vi "validate.vi"(8 "error in":errorcluster, 11 "fixed channel configuration in":refnum<class "control module configuration.lvclass">) -> (0 "error out":errorcluster, 3 "fixed channel configuration out":refnum<class "control module configuration.lvclass">)   [LabVIEW 2013, in "control module configuration.lvclass"]
doc: "This function performs validation of the configuration. This function should be safe to call at any point and should not rely on anything in the runtime environment."
uses:
  control module configuration.lvclass
  <vilib>/NI/Tag Bus Module Framework/module configuration/TBM module configuration.lvclass
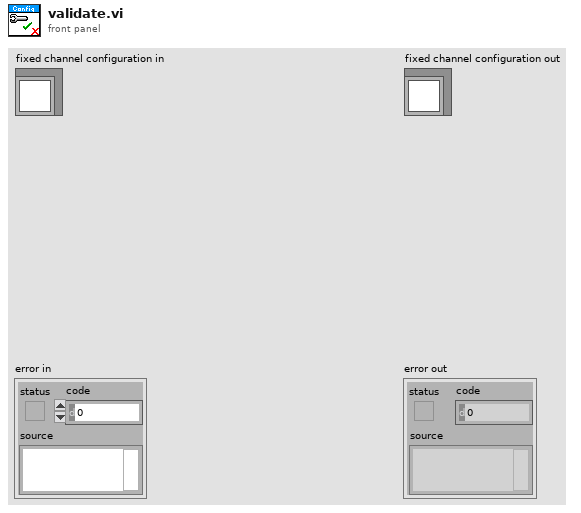
[diagram p1: front panel]
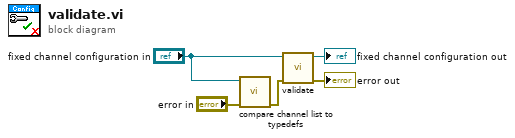
[diagram p0: block diagram]
diagram:
  n1 = call "compare channel list to typedefs.vi"("error in"="error in", "fixed channel configuration"="fixed channel configuration in") -> ("error out"=w3:errorcluster)  [unwired: 9 in]
  n2 = call-parent "validate.vi"("error in"=w3, "configuration in"="fixed channel configuration in") -> ("error out"=→"error out":errorcluster, "configuration out"=→"fixed channel configuration out":refnum<class "control module configuration.lvclass">)  [unwired: 8 in]
